vi "Write Name.vi"(8 "error in (no error)":errorcluster, 10 "Name":string, 11 "Block in":refnum<class "Block.lvclass">) -> (0 "error out":errorcluster, 3 "Block out":refnum<class "Block.lvclass">)   [LabVIEW 2016, in "Block.lvclass"]
uses:
  Block.lvclass
  Block.lvclass/Block.ctl
  Gradient Rectangle/Gradient Rectangle.lvclass
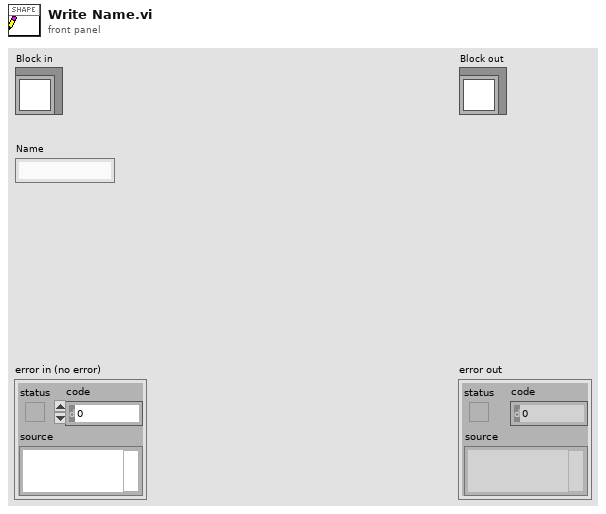
[diagram p1: front panel]
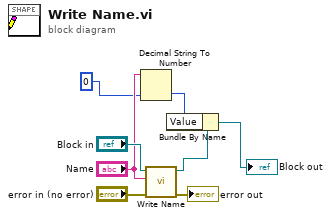
[diagram p0: block diagram]
diagram:
  n1 = Decimal String To Number(string="Name", default (0L)=u32 0) -> (number=w2:u32)  [unwired: 1 in, 1 out]
  n2 = call-parent "Write Name.vi"("error in (no error)"="error in (no error)", "Name"="Name", "Shape in"="Block in") -> ("error out"=→"error out":errorcluster, "Shape out"=w5:refnum<class "Block.lvclass">)  [unwired: 7 in]
  n3 = Bundle By Name(cluster=w5, "Value"=w2) -> (→"Block out":refnum<class "Block.lvclass">)
